vi "Water_Reservoir.vi"() -> ()   [LabVIEW 2020]
panel:
  in  "stop":bool
  out "LED 2":bool
  out "LED 1":bool
  out "Water Reservoir":dbl(slide) scale=0.0..110.0
  in  "D2":dbl(slide) scale=0.0..152.0
  in  "D1":dbl(slide) scale=0.0..120.0
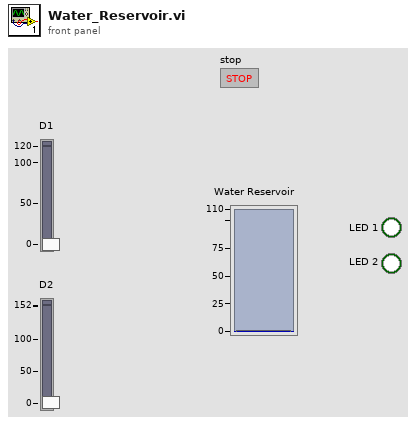
[diagram p1: front panel]
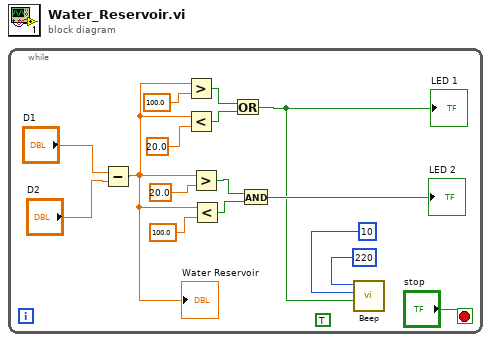
[diagram p0: block diagram]
diagram:
  n1 = while {
    stop <- "stop" stop-if-true
    (unwired) TRUE ("use system alert? (T)")
    n2 = Subtract(x="D1", y="D2") -> (x-y=w11:dbl)
    "Water Reservoir" <- w11
    n3 = Greater?(x=w11, y=100.0) -> (0:w5:bool)
    n4 = Less?(x=w11, y=20.0) -> (x < y?=w6:bool)
    n5 = Greater?(x=w11, y=20.0) -> (0:w7:bool)
    n6 = Less?(x=w11, y=100.0) -> (x < y?=w8:bool)
    n7 = Or(x=w5, y=w6) -> (x .or. y?=w1:bool)
    "LED 1" <- w1
    n8 = And(x=w7, y=w8) -> (x .and. y?=→"LED 2":bool)
    n9 = call <vilib>:"Beep.vi"("use system alert? (T)"=w1, "duration (msec)"=u32 10, "frequency (Hz)"=u32 220) -> ()  [unwired: 9 in]
  }
